vi "sv_Design Fractional Octave Filter.vi"(0 "bandwidth":T3(ring), 1 "standard":T4=enum."IEC 61260", 5 "sampling frequency [Hz]":dbl=10000.0 format="%.2f", 7 "midband frequency [Hz]":dbl=1000.0, 11 "error in (no error)":errorcluster, 12 "coerce to nearest standard midband frequency?":bool) -> (4 "nominal frequencies [Hz]":dbl[](array[numeric]), 6 "filter bank parameters":T1={"octave filter coefficients"=[{"filter structure"=enum."IIR 2nd Order", "Reverse Coefficients"=[1.0], "Forward Coefficients"=[]}], "lowpass filter coefficients"={"filter structure"=enum."IIR 2nd Order", "Reverse Coefficients"=[], "Forward Coefficients"=[]}, "number of samples to settle"=0, "number of decimation steps required"=[], "octave filter bandwidth"=[]}, 8 "initial filter state":T2, 10 "actual midband frequency [Hz]":dbl, 15 "error out":errorcluster)   [LabVIEW 2017, in "SoundVib_Octave_2014 standard.lvlib"]
doc: "This VI designs a single octave filter based on the specified midband frequency and bandwidth.\n\nThe fractional-octave filter is designed in accordance with one of the following standards:\n ANSI S1.11-2014;\n IEC 61260-1:2014.\nFor both standards, the sampling frequency must be at least 3 times the highest midband frequency for octave analysis and at least 2.5 times the highest midband frequency for 1/3, 1/6, 1/12, or 1/24 octave analysis. Available bandwidths are 1/1, 1/3, 1/6, 1/12, and 1/24 octave.\n\nTo design a standard octave filter, set coerce to nearest standard midband frequency to TRUE."
uses:
  <vilib>/addons/Sound and Vibration/svt_Octave/SoundVib_Octave_2014 standard.lvlib
  <vilib>/addons/_NISVFA/_Shared subVIs/Controls/svc_Octave Standard.ctl
  <vilib>/addons/_NISVFA/_Shared subVIs/Controls/svc_Octave Filter State.ctl
  <vilib>/addons/_NISVFA/_Shared subVIs/Controls/svc_Octave Filter Bank Parameters.ctl
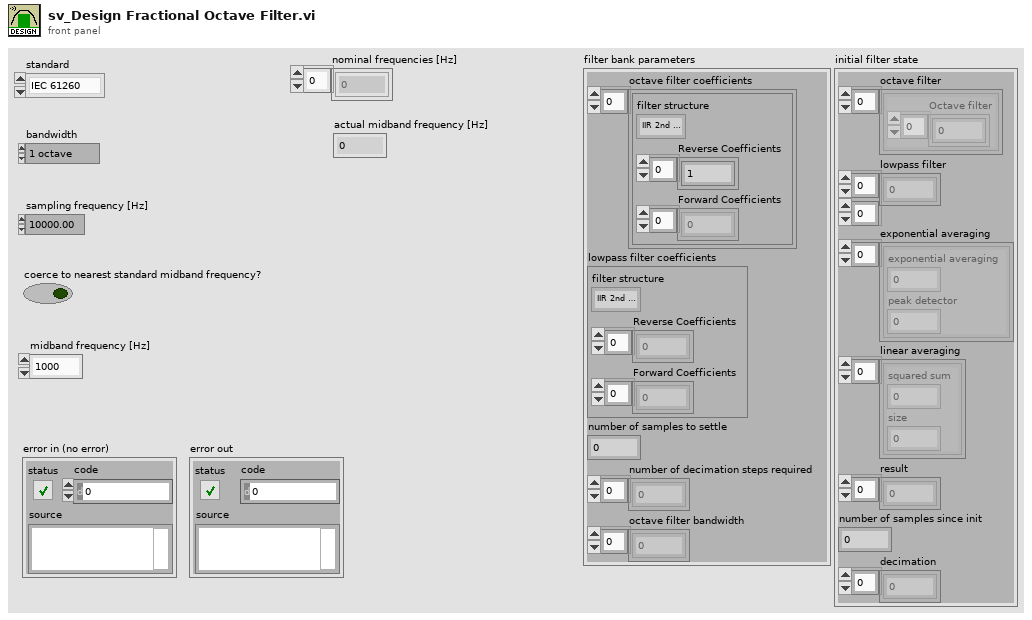
[diagram p1: front panel]
types:
  T1 = typedef "svc_Octave Filter Bank Parameters.ctl" = cluster{"octave filter coefficients":cluster{"filter structure":enum32{"IIR 2nd Order", "IIR 4th Order"}, "Reverse Coefficients":dbl[], "Forward Coefficients":dbl[]}[], "lowpass filter coefficients":cluster{"filter structure":enum32{"IIR 2nd Order", "IIR 4th Order"}, "Reverse Coefficients":dbl[], "Forward Coefficients":dbl[]}, "number of samples to settle":u64, "number of decimation steps required":i32[], "octave filter bandwidth":dbl[]}
  T2 = typedef "svc_Octave Filter State.ctl" = cluster{"octave filter":cluster{"Octave filter":dbl[]}[], "lowpass filter":dbl[][], "exponential averaging":cluster{"exponential averaging":dbl, "peak detector":dbl}[], "linear averaging":cluster{"squared sum":dbl, "size":dbl}[], "result":dbl[], "number of samples since init":u64, "decimation":dbl[]}
  T3 = enum16{"1 octave", "1/3 octave", "1/6 octave", "1/12 octave", "1/24 octave"}
  T4 = typedef "svc_Octave Standard.ctl" = enum16{"ANSI S1.11", "IEC 61260"}
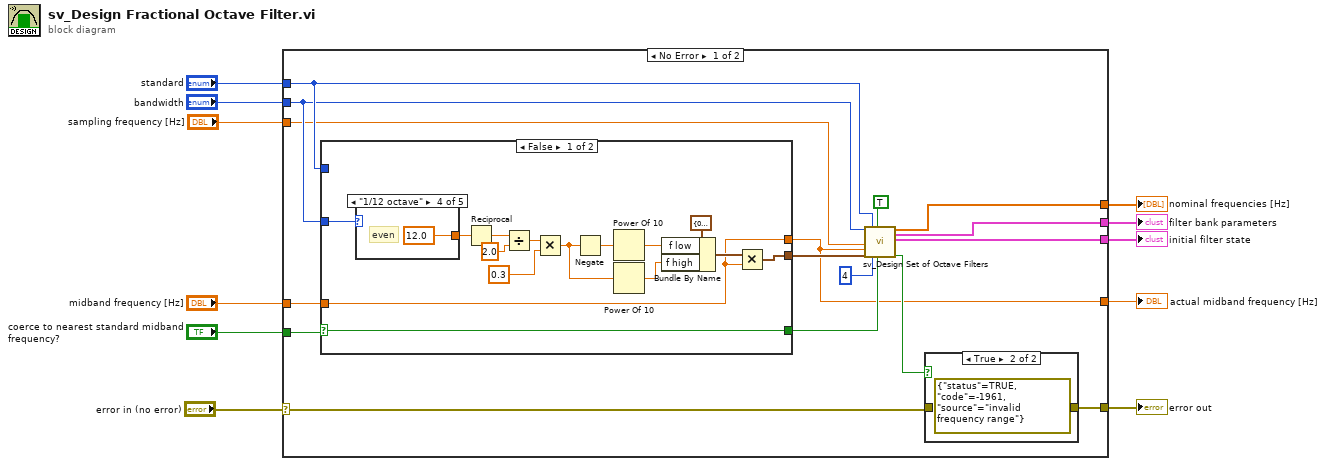
[diagram p0: block diagram]
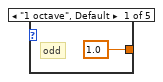
[diagram p3: hidden frame]
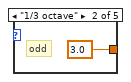
[diagram p4: hidden frame]
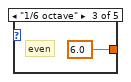
[diagram p5: hidden frame]
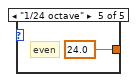
[diagram p6: hidden frame]
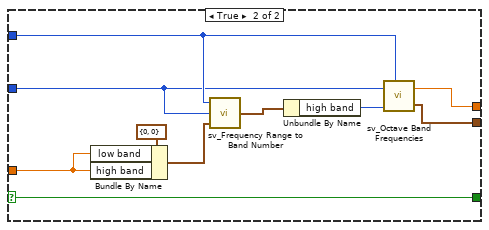
[diagram p7: hidden frame]
diagram:
  n1 = case shown="No Error" "error in (no error)" {
    selector: "error in (no error)" -> [w14 w60]
    tunnel: "coerce to nearest standard midband frequency?" -> [w27 _]
    tunnel: "midband frequency [Hz]" -> [w26 _]
    tunnel: "standard" -> [w23 _]
    tunnel: "bandwidth" -> [w22 _]
    tunnel: "sampling frequency [Hz]" -> [w21 _]
    tunnel: [w18 _] -> w6
    tunnel: [w17 _] -> w5
    tunnel: [w15 _] -> w4
    tunnel: [w13 w60] -> w2
    tunnel: [w12 _] -> w1
    frame No Error {
      n2 = case shown="False" w27 {
        selector: w27 -> [w30 w50]
        tunnel: w26 -> [w33 w55]
        tunnel: w22 -> [w31 w53]
        tunnel: w23 -> [_ w54]
        tunnel: [w33 w52] -> w12
        tunnel: [w32 w51] -> w25
        tunnel: [w30 w50] -> w24
        frame False {
          n3 = case shown="\"1/12 octave\"" w31 {
            tunnel: [1.0 ("x") 3.0 ("x") 6.0 ("x") 12.0 ("x") 24.0 ("x")] -> w34
            frame "1 octave", Default {
              # "odd"
            }
            frame "1/3 octave" {
              # "odd"
            }
            frame "1/6 octave" {
              # "even"
            }
            frame "1/12 octave" {
              # "even"
            }
            frame "1/24 octave" {
              # "even"
            }
          }
          n4 = Reciprocal(x=w34) -> (1/x=w37:dbl)
          n5 = Divide(x=w37, y=2.0) -> (x/y=w36:dbl)
          n6 = Multiply(x=w36, y=0.3) -> (x*y=w40:dbl)
          n7 = Negate(x=w40) -> (-x=w39:dbl)
          n8 = Power Of 10(x=w39) -> (10^x=w42:dbl)
          n9 = Power Of 10(x=w40) -> (10^x=w43:dbl)
          n10 = Bundle By Name(cluster=cluster{"f low":dbl, "f high":dbl} {"f low"=0.0, "f high"=0.0} ("bandedge frequencies [Hz] 2"), "f low"=w42, "f high"=w43) -> (w44:cluster{"f low":dbl, "f high":dbl})
          n11 = Multiply(x=w44, y=w33) -> (x*y=w32:cluster{"f low":dbl, "f high":dbl})
        }
        frame True {
          n12 = Bundle By Name(cluster=cluster{"low band":i32, "high band":i32} {"low band"=0, "high band"=0} ("band number"), "low band"=w55, "high band"=w55) -> (w56:cluster{"low band":i32, "high band":i32})
          n13 = call <vilib>:"sv_Frequency Range to Band Number.vi"("frequency range [Hz]"=w56, "bandwidth"=w53, "standard"=w54) -> ("band number"=w57:cluster{"low band":i32, "high band":i32})
          n14 = Unbundle By Name(w57) -> ("high band"=w58:i32)
          n15 = call <vilib>:"sv_Octave Band Frequencies.vi"("octave band selector"=w58, "bandwidth"=w53, "standard"=w54) -> ("bandedge frequencies [Hz]"=w51:cluster{"f low":dbl, "f high":dbl}, "midband frequency [Hz]"=w52:dbl)  [unwired: 1 in, 2 out]
        }
      }
      n16 = call <vilib>:"sv_Design Set of Octave Filters.vi"("bandwidth"=w22, "sampling frequency [Hz]"=w21, "adjusted midband frequency [Hz]"=w12, "adjusted bandedge frequencies [Hz]"=w25, "standard"=w23, "Butterworth filter order"=4, "band specified by midband frequency?"=TRUE, "Is filter standard?"=w24) -> ("nominal frequencies [Hz]"=w15:dbl[], "filter bank parameters"=w17:T1, "initialize filter state"=w18:T2, "error"=w16:bool)  [unwired: 6 in, 2 out]
      n17 = case shown="True" w16 {
        tunnel: w14 -> [w28 _]
        tunnel: [w28 errorcluster {"status"=TRUE, "code"=-1961, "source"="invalid frequency range"} ("error IO")] -> w13
        frame False {
        }
        frame True {
        }
      }
    }
    frame Error {
    }
  }
  "initial filter state" <- w6
  "filter bank parameters" <- w5
  "nominal frequencies [Hz]" <- w4
  "error out" <- w2
  "actual midband frequency [Hz]" <- w1
